vi "Enable Controllers.vi"() -> ()   [LabVIEW 2018]
panel:
  out "appended array 2":dbl[](array[numeric])
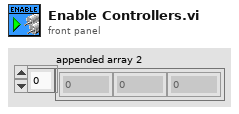
[diagram p1: front panel]
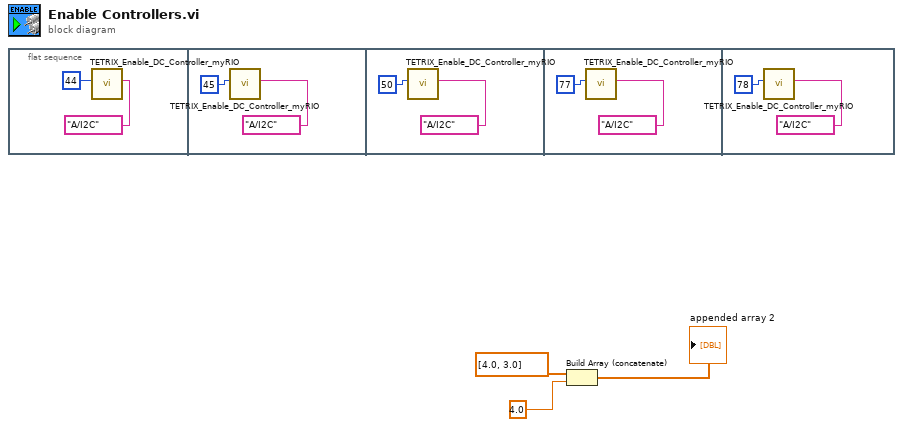
[diagram p0: block diagram]
diagram:
  n1 = flat-sequence {
    frame #0 {
      n2 = call <vilib>:"TETRIX_Enable_DC_Controller_myRIO.vi"("myRIO MXP Port A/B"=tag "A/I2C", "Controller ID#  (I2C Address)"=u8 44) -> ()  [unwired: 5 in, 1 out]
    }
    frame #1 {
      n3 = call <vilib>:"TETRIX_Enable_DC_Controller_myRIO.vi"("myRIO MXP Port A/B"=tag "A/I2C", "Controller ID#  (I2C Address)"=u8 45) -> ()  [unwired: 5 in, 1 out]
    }
    frame #2 {
      n4 = call <vilib>:"TETRIX_Enable_DC_Controller_myRIO.vi"("myRIO MXP Port A/B"=tag "A/I2C", "Controller ID#  (I2C Address)"=u8 50) -> ()  [unwired: 5 in, 1 out]
    }
    frame #3 {
      n5 = call <vilib>:"TETRIX_Enable_DC_Controller_myRIO.vi"("myRIO MXP Port A/B"=tag "A/I2C", "Controller ID#  (I2C Address)"=u8 77) -> ()  [unwired: 5 in, 1 out]
    }
    frame #4 {
      n6 = call <vilib>:"TETRIX_Enable_DC_Controller_myRIO.vi"("myRIO MXP Port A/B"=tag "A/I2C", "Controller ID#  (I2C Address)"=u8 78) -> ()  [unwired: 5 in, 1 out]
    }
  }
  n7 = Build Array (concatenate)(dbl[] [4.0, 3.0] ("array"), 4.0 ("element")) -> (→"appended array 2":dbl[])
